vi "file control panel.vi"() -> ()   [LabVIEW 2017]
uses:
  control panel globals.vi
panel:
  out "error out":errorcluster
  in  "open files":bool
  out "elements in queues":T1
  in  "close files":bool
  out "time stamp (write in your lab book)":string
  out "data directory":path
  in  "set data dir":bool
  in  "clear \nstored":bool
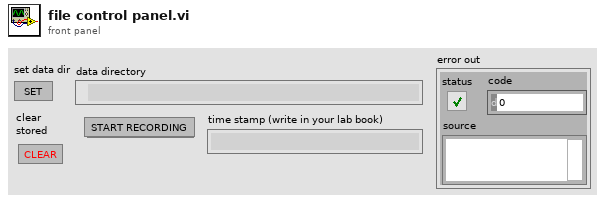
[diagram p1: front panel]
types:
  T1 = cluster{"voltage":i32, "coil":i32, "mag":i32, "accel":i32}
  T2 = typedef "queue cluster.ctl" = cluster{"voltage":T3, "coil":T3, "mag":T3, "accel":T3, "slope":refnum<queue>, "angle":refnum<queue>}
  T3 = typedef "reading queue.ctl" = refnum<queue>
  T4 = cluster{refnum<k0>, refnum<k0>, refnum<k0>, refnum<k0>, refnum<k0>}
  T5 = typedef "refnum cluster.ctl" = cluster{"voltage file":refnum<file>, "coil file":refnum<file>, "mag file":refnum<file>, "slope file":refnum<file>, "angle file":refnum<file>}
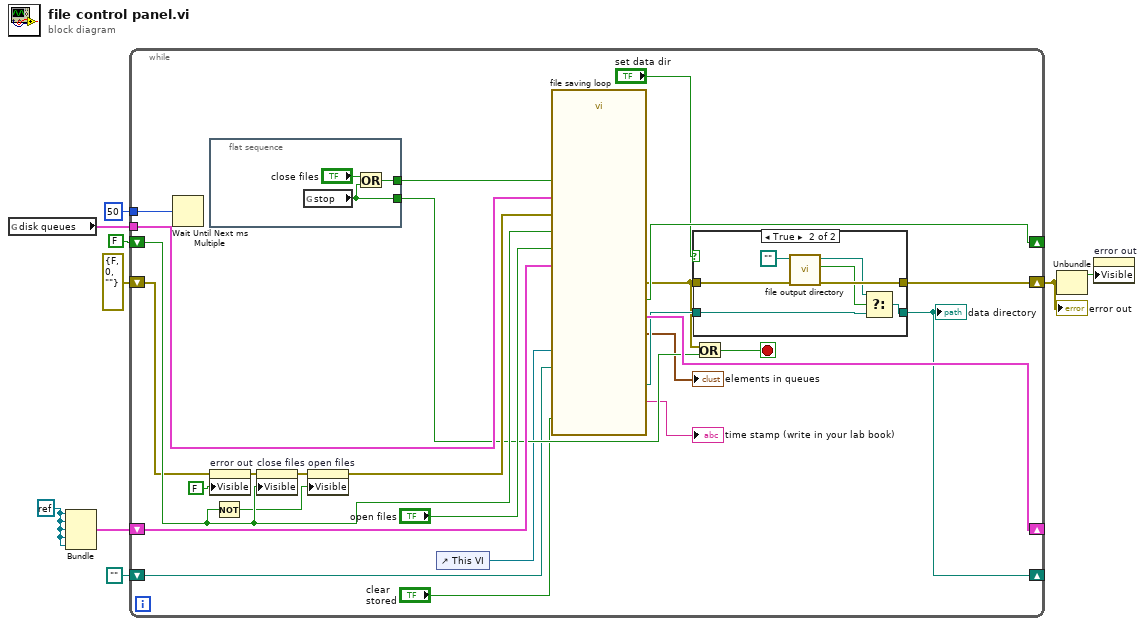
[diagram p0: block diagram]
diagram:
  w8 = refnum<k0> refnum
  n1 = global read "control panel globals.vi" "disk queues"() -> (w9:T2)
  n2 = Bundle(w8, w8, w8, w8, w8) -> (w6:T4)  [unwired: 1 in]
  n3 = while {
    tunnel: w9 -> [w34]
    shift-right: [w33] -> _
    shift-left: FALSE ("files open out") -> [w30]
    shift-right: [w15] -> w2
    shift-left: errorcluster {"status"=FALSE, "code"=0, "source"=""} ("error out") -> [w12]
    shift-right: [w28] -> _
    shift-left: w6 -> [w27]
    tunnel: i64 50 ("update (ms)") -> [w22]
    shift-right: [w17] -> _
    shift-left: path "" -> [w21]
    stop <- w26 stop-if-true
    n4 = Wait Until Next ms Multiple(millisecond multiple=w22) -> ()  [unwired: 1 out]
    n5 = flat-sequence {
      tunnel: [w46] -> w25
      tunnel: [w45] -> w24
      frame #0 {
        n6 = global read "control panel globals.vi" "stop"() -> (w45:bool)
        n7 = Or(x="close files", y=w45) -> (x .or. y?=w46:bool)
      }
    }
    n8 = property on="error out" class="Clust (strict)"(error in=w12, "Visible"=FALSE) -> (error out=w11:errorcluster)  [unwired: 1 in, 1 out]
    n9 = Not(x=w30) -> (.not. x?=w29:bool)
    n10 = property on="close files" class="Bool"(error in=w11, "Visible"=w30) -> (error out=w32:errorcluster)  [unwired: 1 in, 1 out]
    n11 = property on="open files" class="Bool"(error in=w32, "Visible"=w29) -> (error out=w31:errorcluster)  [unwired: 1 in, 1 out]
    n12 = control-ref of="This VI"() -> (w23:refnum<vi>)
    n13 = call "file saving loop.vi"("files open"=w30, "refnums"=w27, "disk queues"=w34, "close files"=w25, "open files"="open files", "error in"=w31, "clear"="clear \nstored", "data directory in"=w21, "main vi ref"=w23) -> ("data directory"=w18:path, "files open out"=w33:bool, "refnums out"=w28:T5, "time stamp (write in your lab book)"=→"time stamp (write in your lab book)":string, "elements in queues"=→"elements in queues":T1, "error out"=w16:errorcluster)  [unwired: 5 in]
    n14 = case shown="True" "set data dir" {
      tunnel: w18 -> [w37 w39]
      tunnel: [w37 w40] -> w17
      tunnel: w16 -> [w36 w44]
      tunnel: [w36 w43] -> w15
      frame False {
      }
      frame True {
        n15 = call "file output directory.vi"("error in"=w44, "data directory in"=path "") -> ("error out"=w43:errorcluster, "exists"=w42:bool, "data directory"=w41:path)  [unwired: 7 in]
        n16 = Select(t=w41, s=w42, f=w39) -> (s? t:f=w40:path)
      }
    }
    "data directory" <- w17
    n17 = Or(x=w16, y=w24) -> (x .or. y?=w26:bool)
  }
  "error out" <- w2
  n18 = Unbundle(w2) -> ("status"=w1:bool)  [unwired: 2 out]
  n19 = property on="error out" class="Clust (strict)"("Visible"=w1) -> ()  [unwired: 2 in, 2 out]
